vi "serpConfig.vi"() -> ()   [LabVIEW 2020]
doc: "This VI was removed from the Functions palette. Use the VIs and functions on the VISA palette to control serial devices. If you use the LabVIEW PDA Module, use this VI for serial communication."
panel:
  in  "VISA Aliases":string[](array[string])
  in  "delay break ?":bool=TRUE
  in  "specific reset ?":bool=TRUE
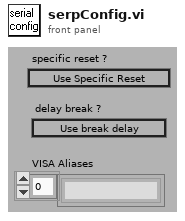
[diagram p1: front panel]
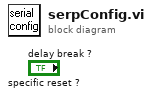
[diagram p0: block diagram]
diagram:
